vi "DAQ Configuration Validation.vi"(4 "Maximum Value":dbl, 5 "DAQ Resource Name":string, 6 "Minimum Value":dbl, 7 "Sensor Type":T1, 8 "error in":errorcluster, 9 "scale type":variant, 10 "scaling info":variant, 11 "bridge info":variant) -> (0 "error IO":errorcluster, 2 "Error Source":string, 3 "Valid configuration?":bool)   [LabVIEW 2010, in "PXIe-433x Custom Device.lvlib"]
uses:
  PXIe-433x Custom Device.lvlib
  Sensor Type.ctl
  Strain Bridge Information.ctl
  Strain Information.ctl
  Scale Type.ctl
  <vilib>/Utility/error.llb/DialogType.ctl
  <vilib>/DAQmx/configure/timing.llb/DAQmx Timing (Sample Clock).vi
  <vilib>/DAQmx/create/channels.llb/DAQmx Create Channel (AI-Strain-Strain Gage).vi
  <vilib>/DAQmx/create/channels.llb/DAQmx Create Channel (AI-Force-Bridge-Two-Point-Linear).vi
  <vilib>/DAQmx/create/channels.llb/DAQmx Create Channel (AI-Force-Bridge-Table).vi
  <vilib>/DAQmx/create/channels.llb/DAQmx Create Channel (AI-Force-Bridge-Polynomial).vi
  <vilib>/DAQmx/create/channels.llb/DAQmx Create Channel (AI-Pressure-Bridge-Two-Point-Linear).vi
  <vilib>/DAQmx/create/channels.llb/DAQmx Create Channel (AI-Pressure-Bridge-Table).vi
  <vilib>/DAQmx/create/channels.llb/DAQmx Create Channel (AI-Pressure-Bridge-Polynomial).vi
  <vilib>/DAQmx/create/channels.llb/DAQmx Create Channel (AI-Torque-Bridge-Two-Point-Linear).vi
  <vilib>/DAQmx/create/channels.llb/DAQmx Create Channel (AI-Torque-Bridge-Table).vi
  <vilib>/DAQmx/create/channels.llb/DAQmx Create Channel (AI-Torque-Bridge-Polynomial).vi
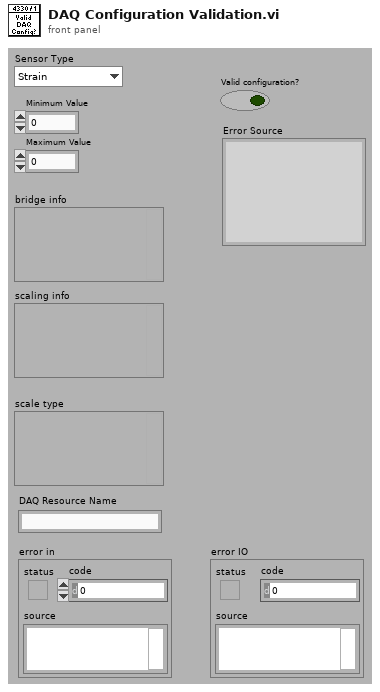
[diagram p1: front panel]
types:
  T1 = typedef "PXIe-433x Custom Device.lvlib/Sensor Type.ctl" = enum16{"Strain", "Force", "Pressure", "Torque"}
  T2 = typedef "PXIe-433x Custom Device.lvlib/Strain Bridge Information.ctl" = cluster{"strain configuration":i32, "lead wire resistance":dbl, "initial bridge voltage":dbl, "voltage excitation source":i32, "voltage excitation value":dbl}
  T3 = typedef "PXIe-433x Custom Device.lvlib/Strain Information.ctl" = cluster{"gage factor":dbl, "nominal gage resistance":dbl, "poisson ratio":dbl}
  T4 = cluster{"bridge configuration":i32, "voltage excitation source":i32, "voltage excitation value":dbl, "nominal bridge resistance":dbl}
  T5 = typedef "PXIe-433x Custom Device.lvlib/Scale Type.ctl" = enum16{"Linear", "Table", "Polynomial"}
  T6 = cluster{"first electrical value":dbl, "second electrical value":dbl, "electrical units":i32, "first physical value":dbl, "second physical value":dbl, "physical units":i32}
  T7 = cluster{"electrical values":dbl[], "electrical units":i32, "physical values":dbl[], "physical units":i32}
  T8 = cluster{"forward coeff":dbl[], "reverse coeff":dbl[], "electrical units":i32, "physical units":i32}
  T9 = typedef "DialogType.ctl" = u16
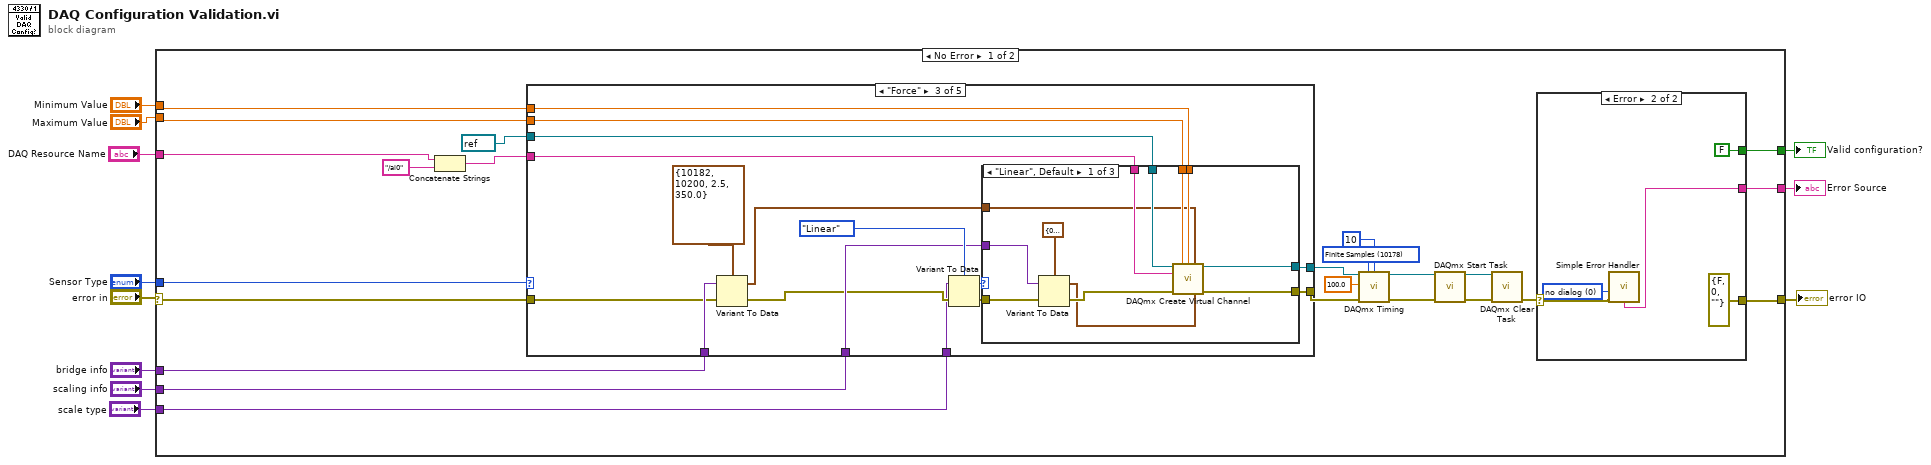
[diagram p0: block diagram]
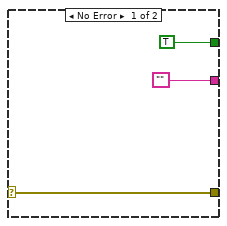
[diagram p2: hidden frame]
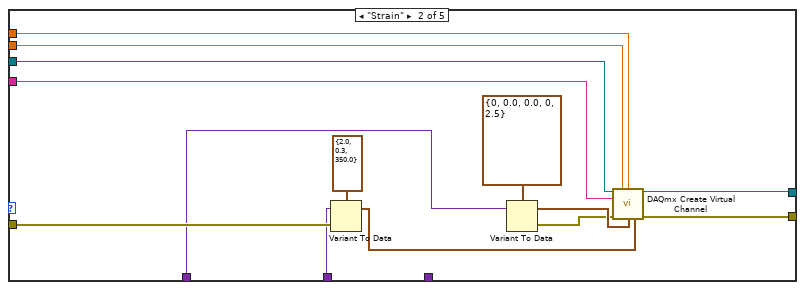
[diagram p4: hidden frame]
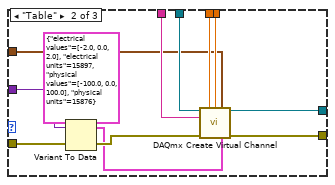
[diagram p5: hidden frame]
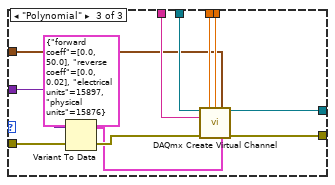
[diagram p6: hidden frame]
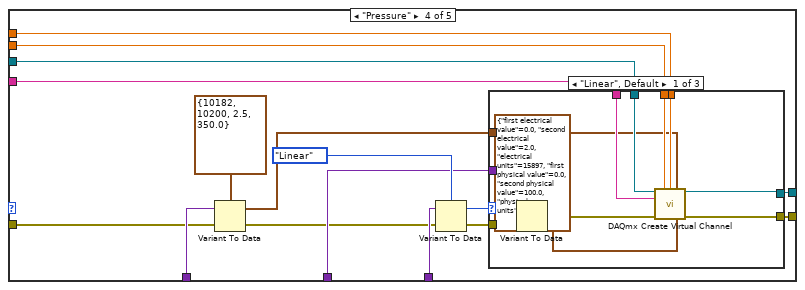
[diagram p7: hidden frame]
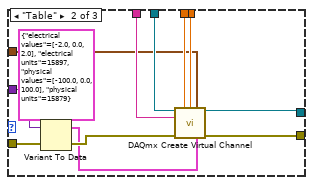
[diagram p8: hidden frame]
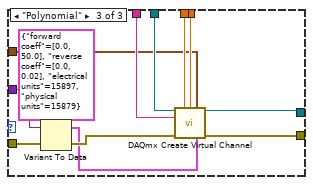
[diagram p9: hidden frame]
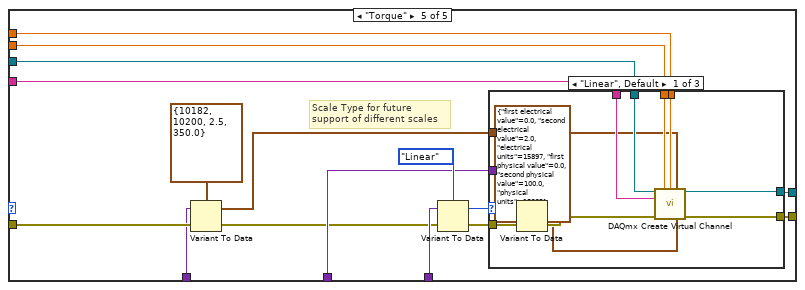
[diagram p10: hidden frame]
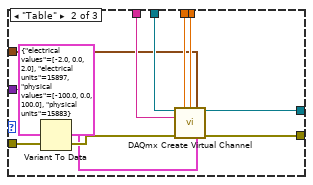
[diagram p11: hidden frame]
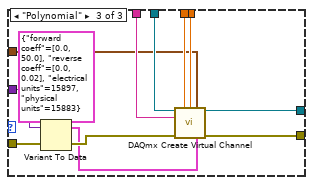
[diagram p12: hidden frame]
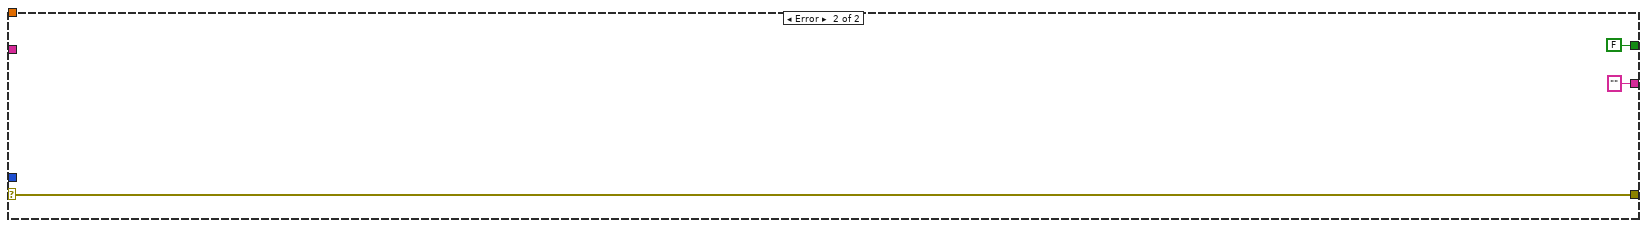
[diagram p13: hidden frame]
diagram:
  n1 = case shown="No Error" "error in" {
    selector: "error in" -> [w25 w218]
    tunnel: [w15 w218] -> w2
    tunnel: "Sensor Type" -> [w31 _]
    tunnel: "Minimum Value" -> [w30 _]
    tunnel: "Maximum Value" -> [w29 _]
    tunnel: "scale type" -> [w28 _]
    tunnel: "scaling info" -> [w27 _]
    tunnel: "bridge info" -> [w26 _]
    tunnel: [w14 FALSE] -> w10
    tunnel: [w13 "" ("source")] -> w11
    tunnel: "DAQ Resource Name" -> [w12 _]
    frame No Error {
      w20 = 10178 items=["Finite Samples"=10178, "Continuous Samples"=10123, "Hardware Timed Single Point"=12522] ("sample mode")
      n2 = Concatenate Strings(w12, "/ai0" ("string")) -> (w33:string)
      n3 = case shown="\"Force\"" w31 {
        tunnel: [w44 w59 w75 w127 w179] -> w34
        tunnel: refnum<k21> refnum ("task out") -> [w44 w58 w74 w126 w178]
        tunnel: w33 -> [_ w57 w73 w125 w177]
        tunnel: [w45 w56 w72 w124 w176] -> w23
        tunnel: w25 -> [w45 w48 w63 w115 w168]
        tunnel: w30 -> [_ w51 w70 w122 w174]
        tunnel: w29 -> [_ w50 w69 w121 w173]
        tunnel: w26 -> [_ w46 w64 w116 w167]
        tunnel: w27 -> [_ w47 w62 w113 w165]
        tunnel: w28 -> [_ _ w60 w114 w166]
        frame Default {
        }
        frame "Strain" {
          n4 = Variant To Data(error in=w48, Variant=w47, type=T3 {"gage factor"=2.0, "nominal gage resistance"=0.3, "poisson ratio"=350.0} ("strain gage information")) -> (data=w53:T3)  [unwired: 1 out]
          n5 = Variant To Data(Variant=w46, type=T2 {"strain configuration"=0, "lead wire resistance"=0.0, "initial bridge voltage"=0.0, "voltage excitation source"=0, "voltage excitation value"=2.5} ("bridge information")) -> (error out=w52:errorcluster, data=w54:T2)  [unwired: 1 in]
          n6 = call-poly <vilib>:"DAQmx Create Virtual Channel.vi"("task in"=w58, "maximum value"=w50, "minimum value"=w51, "physical channels"=w57, "error in"=w52, "bridge information"=w54, "strain gage information"=w53) -> ("task out"=w59:refnum<k21>, "error out"=w56:errorcluster)  [unwired: 7 in]
        }
        frame "Force" {
          n7 = Variant To Data(error in=w63, Variant=w64, type=T4 {"bridge configuration"=10182, "voltage excitation source"=10200, "voltage excitation value"=2.5, "nominal bridge resistance"=350.0} ("bridge information")) -> (error out=w61:errorcluster, data=w68:T4)
          n8 = Variant To Data(error in=w61, Variant=w60, type=Scale_Type."Linear" ("Scale Type")) -> (error out=w71:errorcluster, data=w67:T5)
          n9 = case shown="\"Linear\", Default" w67 {
            tunnel: [w87 w99 w111] -> w75
            tunnel: w74 -> [w86 w98 w110]
            tunnel: w73 -> [w85 w97 w109]
            tunnel: [w84 w96 w108] -> w72
            tunnel: w71 -> [w80 w92 w104]
            tunnel: w70 -> [w83 w95 w107]
            tunnel: w69 -> [w82 w94 w106]
            tunnel: w68 -> [w81 w93 w105]
            tunnel: w62 -> [w78 w90 w102]
            frame "Linear", Default {
              n10 = Variant To Data(error in=w80, Variant=w78, type=T6 {"first electrical value"=0.0, "second electrical value"=2.0, "electrical units"=15897, "first physical value"=0.0, "second physical value"=100.0, "physical units"=15876} ("scaling information")) -> (error out=w79:errorcluster, data=w76:T6)
              n11 = call-poly <vilib>:"DAQmx Create Virtual Channel.vi"("task in"=w86, "maximum value"=w82, "minimum value"=w83, "bridge information"=w81, "physical channels"=w85, "error in"=w79, "scaling information"=w76) -> ("task out"=w87:refnum<k21>, "error out"=w84:errorcluster)  [unwired: 7 in]
            }
            frame "Table" {
              n12 = Variant To Data(error in=w92, Variant=w90, type=T7 {"electrical values"=[-2.0, 0.0, 2.0], "electrical units"=15897, "physical values"=[-100.0, 0.0, 100.0], "physical units"=15876} ("scaling information")) -> (error out=w91:errorcluster, data=w89:T7)
              n13 = call-poly <vilib>:"DAQmx Create Virtual Channel.vi"("task in"=w98, "maximum value"=w94, "minimum value"=w95, "bridge information"=w93, "physical channels"=w97, "error in"=w91, "scaling information"=w89) -> ("task out"=w99:refnum<k21>, "error out"=w96:errorcluster)  [unwired: 7 in]
            }
            frame "Polynomial" {
              n14 = Variant To Data(error in=w104, Variant=w102, type=T8 {"forward coeff"=[0.0, 50.0], "reverse coeff"=[0.0, 0.02], "electrical units"=15897, "physical units"=15876} ("scaling information")) -> (error out=w103:errorcluster, data=w101:T8)
              n15 = call-poly <vilib>:"DAQmx Create Virtual Channel.vi"("task in"=w110, "maximum value"=w106, "minimum value"=w107, "bridge information"=w105, "physical channels"=w109, "error in"=w103, "scaling information"=w101) -> ("task out"=w111:refnum<k21>, "error out"=w108:errorcluster)  [unwired: 7 in]
            }
          }
        }
        frame "Pressure" {
          n16 = Variant To Data(error in=w115, Variant=w116, type=T4 {"bridge configuration"=10182, "voltage excitation source"=10200, "voltage excitation value"=2.5, "nominal bridge resistance"=350.0} ("bridge information")) -> (error out=w112:errorcluster, data=w120:T4)
          n17 = Variant To Data(error in=w112, Variant=w114, type=Scale_Type."Linear" ("Scale Type")) -> (error out=w123:errorcluster, data=w119:T5)
          n18 = case shown="\"Linear\", Default" w119 {
            tunnel: [w139 w151 w163] -> w127
            tunnel: w126 -> [w138 w150 w162]
            tunnel: w125 -> [w137 w149 w161]
            tunnel: [w136 w148 w160] -> w124
            tunnel: w123 -> [w132 w144 w156]
            tunnel: w122 -> [w135 w147 w159]
            tunnel: w121 -> [w134 w146 w158]
            tunnel: w120 -> [w133 w145 w157]
            tunnel: w113 -> [w130 w142 w154]
            frame "Linear", Default {
              n19 = Variant To Data(error in=w132, Variant=w130, type=T6 {"first electrical value"=0.0, "second electrical value"=2.0, "electrical units"=15897, "first physical value"=0.0, "second physical value"=100.0, "physical units"=15879} ("scaling information")) -> (error out=w131:errorcluster, data=w129:T6)
              n20 = call-poly <vilib>:"DAQmx Create Virtual Channel.vi"("task in"=w138, "maximum value"=w134, "minimum value"=w135, "bridge information"=w133, "physical channels"=w137, "error in"=w131, "scaling information"=w129) -> ("task out"=w139:refnum<k21>, "error out"=w136:errorcluster)  [unwired: 7 in]
            }
            frame "Table" {
              n21 = Variant To Data(error in=w144, Variant=w142, type=T7 {"electrical values"=[-2.0, 0.0, 2.0], "electrical units"=15897, "physical values"=[-100.0, 0.0, 100.0], "physical units"=15879} ("scaling information")) -> (error out=w143:errorcluster, data=w141:T7)
              n22 = call-poly <vilib>:"DAQmx Create Virtual Channel.vi"("task in"=w150, "maximum value"=w146, "minimum value"=w147, "bridge information"=w145, "physical channels"=w149, "error in"=w143, "scaling information"=w141) -> ("task out"=w151:refnum<k21>, "error out"=w148:errorcluster)  [unwired: 7 in]
            }
            frame "Polynomial" {
              n23 = Variant To Data(error in=w156, Variant=w154, type=T8 {"forward coeff"=[0.0, 50.0], "reverse coeff"=[0.0, 0.02], "electrical units"=15897, "physical units"=15879} ("scaling information")) -> (error out=w155:errorcluster, data=w153:T8)
              n24 = call-poly <vilib>:"DAQmx Create Virtual Channel.vi"("task in"=w162, "maximum value"=w158, "minimum value"=w159, "bridge information"=w157, "physical channels"=w161, "error in"=w155, "scaling information"=w153) -> ("task out"=w163:refnum<k21>, "error out"=w160:errorcluster)  [unwired: 7 in]
            }
          }
        }
        frame "Torque" {
          # "Scale Type for future support of different scales"
          n25 = Variant To Data(error in=w168, Variant=w167, type=T4 {"bridge configuration"=10182, "voltage excitation source"=10200, "voltage excitation value"=2.5, "nominal bridge resistance"=350.0} ("bridge information")) -> (error out=w164:errorcluster, data=w172:T4)
          n26 = Variant To Data(error in=w164, Variant=w166, type=Scale_Type."Linear" ("Scale Type")) -> (error out=w175:errorcluster, data=w171:T5)
          n27 = case shown="\"Linear\", Default" w171 {
            tunnel: [w191 w203 w215] -> w179
            tunnel: w178 -> [w190 w202 w214]
            tunnel: w177 -> [w189 w201 w213]
            tunnel: [w188 w200 w212] -> w176
            tunnel: w175 -> [w184 w197 w208]
            tunnel: w174 -> [w187 w199 w211]
            tunnel: w173 -> [w186 w198 w210]
            tunnel: w172 -> [w185 w192 w209]
            tunnel: w165 -> [w182 w195 w206]
            frame "Linear", Default {
              n28 = Variant To Data(error in=w184, Variant=w182, type=T6 {"first electrical value"=0.0, "second electrical value"=2.0, "electrical units"=15897, "first physical value"=0.0, "second physical value"=100.0, "physical units"=15883} ("scaling information")) -> (error out=w183:errorcluster, data=w181:T6)
              n29 = call-poly <vilib>:"DAQmx Create Virtual Channel.vi"("task in"=w190, "maximum value"=w186, "minimum value"=w187, "bridge information"=w185, "physical channels"=w189, "error in"=w183, "scaling information"=w181) -> ("task out"=w191:refnum<k21>, "error out"=w188:errorcluster)  [unwired: 7 in]
            }
            frame "Table" {
              n30 = Variant To Data(error in=w197, Variant=w195, type=T7 {"electrical values"=[-2.0, 0.0, 2.0], "electrical units"=15897, "physical values"=[-100.0, 0.0, 100.0], "physical units"=15883} ("scaling information")) -> (error out=w196:errorcluster, data=w194:T7)
              n31 = call-poly <vilib>:"DAQmx Create Virtual Channel.vi"("task in"=w202, "maximum value"=w198, "minimum value"=w199, "bridge information"=w192, "physical channels"=w201, "error in"=w196, "scaling information"=w194) -> ("task out"=w203:refnum<k21>, "error out"=w200:errorcluster)  [unwired: 7 in]
            }
            frame "Polynomial" {
              n32 = Variant To Data(error in=w208, Variant=w206, type=T8 {"forward coeff"=[0.0, 50.0], "reverse coeff"=[0.0, 0.02], "electrical units"=15897, "physical units"=15883} ("scaling information")) -> (error out=w207:errorcluster, data=w205:T8)
              n33 = call-poly <vilib>:"DAQmx Create Virtual Channel.vi"("task in"=w214, "maximum value"=w210, "minimum value"=w211, "bridge information"=w209, "physical channels"=w213, "error in"=w207, "scaling information"=w205) -> ("task out"=w215:refnum<k21>, "error out"=w212:errorcluster)  [unwired: 7 in]
            }
          }
        }
      }
      n34 = call-poly <vilib>:"DAQmx Timing.vi"("task/channels in"=w34, "sample mode"=w20, "samples per channel"=10, "rate"=100.0, "error in"=w23) -> ("task out"=w24:refnum<k21>, "error out"=w21:errorcluster)  [unwired: 9 in]
      n35 = call <vilib>:"DAQmx Start Task.vi"("task/channels in"=w24, "error in"=w21) -> ("task out"=w22:refnum<k21>, "error out"=w17:errorcluster)  [unwired: 12 in]
      n36 = call <vilib>:"DAQmx Clear Task.vi"("task in"=w22, "error in"=w17) -> ("error out"=w16:errorcluster)  [unwired: 13 in]
      n37 = case shown="Error" w16 {
        selector: w16 -> [w38 w41]
        tunnel: [w38 errorcluster {"status"=FALSE, "code"=0, "source"=""} ("error IO")] -> w15
        tunnel: [TRUE FALSE] -> w14
        tunnel: ["" w39] -> w13
        frame No Error {
        }
        frame Error {
          w40 = T9 0 items=["no dialog", "OK message", "continue or stop message", "OK message + warnings", "continue/stop + warnings"] ("type of dialog (OK msg:1)")
          n38 = call <vilib>:"Simple Error Handler.vi"("type of dialog (OK msg:1)"=w40, "error in (no error)"=w41) -> ("message"=w39:string)  [unwired: 3 in, 4 out]
        }
      }
    }
    frame Error {
    }
  }
  "Error Source" <- w11
  "Valid configuration?" <- w10
  "error IO" <- w2
